vi "Clear.vi"(8 "error in (no error)":errorcluster, 11 "Locus Recorder in":refnum<class "Locus Recorder.lvclass">) -> (0 "error out":errorcluster, 3 "Locus Recorder out":refnum<class "Locus Recorder.lvclass">)   [LabVIEW 2014, in "Locus Recorder.lvclass"]
uses:
  Locus Recorder.lvclass
  Locus Recorder.lvclass/Locus Recorder.ctl
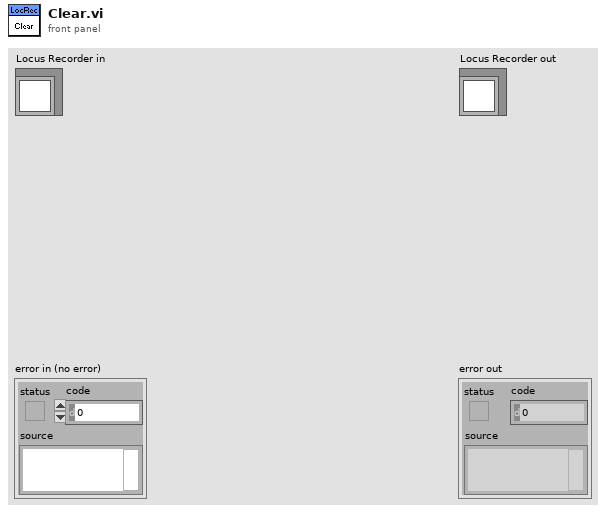
[diagram p1: front panel]
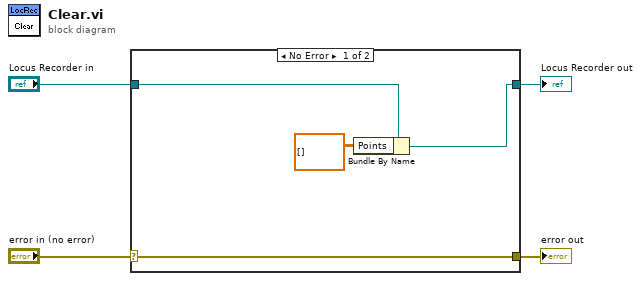
[diagram p0: block diagram]
diagram:
  n1 = case shown="No Error" "error in (no error)" {
    selector: "error in (no error)" -> [w8 w9]
    tunnel: [w8 w9] -> w3
    tunnel: [w5 w10] -> w1
    tunnel: "Locus Recorder in" -> [w7 w10]
    frame No Error {
      n2 = Bundle By Name(cluster=w7, "Points"=dbl[][] []) -> (w5:refnum<class "Locus Recorder.lvclass">)
    }
    frame Error {
    }
  }
  "error out" <- w3
  "Locus Recorder out" <- w1
